vi "PSTR-Replot PSDs.vi"(0 "Data":T1, 2 "Graph Ref":refnum<vi>, 5 "ifreq":i32, 9 "ilevel":i32, 11 "error in (no error)":errorcluster) -> (15 "error out":errorcluster)   [LabVIEW 2020]
uses:
  Typedefs/PSTR-Data.ctl
  Typedefs/PSTR-Model Fit.ctl
  Typedefs/PSTR-Fit Parameters.ctl
  epl-vi-lib/Utility VIs/Conversion VIs/Create Waveform Cluster (1D).vi
panel:
  # "NF x NL x 2 x Npts"
  # "NF x NL x Npts"
  # "NF x NL"
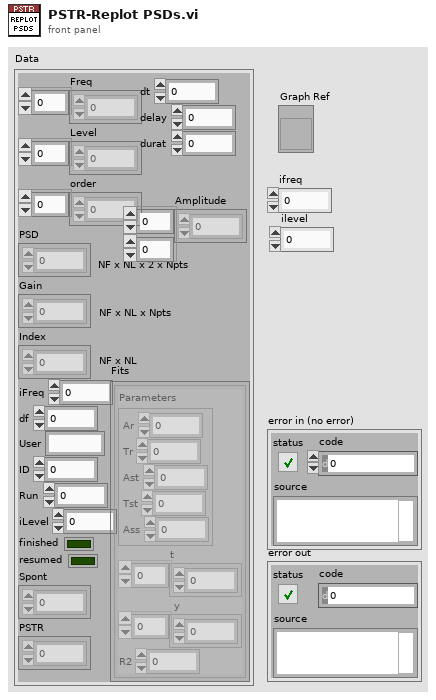
[diagram p1: front panel]
types:
  T1 = typedef "PSTR-Data.ctl" = cluster{"Freq":dbl[], "Level":dbl[], "order":i32[], "PSD":dbl[][][][], "Gain":dbl[][][], "Index":dbl[][], "iFreq":i32, "df":dbl, "User":string, "ID":i32, "Run":i32, "iLevel":i32, "finished":bool, "resumed":bool, "Spont":dbl[][], "PSTR":dbl[][][], "dt":dbl, "delay":dbl, "durat":dbl, "Fits":T2[][], "Amplitude":dbl[][]}
  T2 = typedef "PSTR-Model Fit.ctl" = cluster{"Parameters":T3, "t":dbl[], "y":dbl[], "R2":dbl}
  T3 = typedef "PSTR-Fit Parameters.ctl" = cluster{"Ar":dbl, "Tr":dbl, "Ast":dbl, "Tst":dbl, "Ass":dbl}
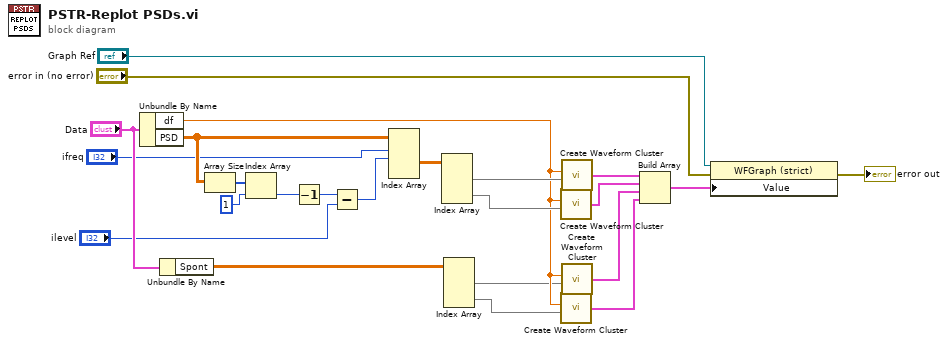
[diagram p0: block diagram]
diagram:
  n1 = Unbundle By Name("Data") -> ("df"=w15:dbl, "PSD"=w17:dbl[][][][])
  n2 = Unbundle By Name("Data") -> ("Spont"=w8:dbl[][])
  n3 = Array Size(array=w17) -> (size(s)=w23:i32[])
  n4 = Index Array(array=w23, index=1) -> (element=w3:i32)
  n5 = Decrement(x=w3) -> (x-1=w6:i32)
  n6 = Subtract(x=w6, y="ilevel") -> (x-y=w4:i32)
  n7 = Index Array(array=w17, index (dim 0)="ifreq", index (dim 1)=w4) -> (element=w22:dbl[][])  [unwired: 2 in]
  n8 = Index Array(array=w22) -> (element #1=w19:dbl[], element #2=w18:dbl[])  [unwired: 4 in]
  n9 = Index Array(array=w8) -> (element #1=w1:dbl[], element #2=w16:dbl[])  [unwired: 4 in]
  n10 = call-poly "Create Waveform Cluster.vi"("dx"=w15, "Y"=w18) -> ("waveform cluster"=w20:cluster{dbl, "dx":dbl, "Y":dbl[]})  [unwired: 3 in]
  n11 = call-poly "Create Waveform Cluster.vi"("dx"=w15, "Y"=w16) -> ("waveform cluster"=w13:cluster{dbl, "dx":dbl, "Y":dbl[]})  [unwired: 3 in]
  n12 = call-poly "Create Waveform Cluster.vi"("dx"=w15, "Y"=w19) -> ("waveform cluster"=w21:cluster{dbl, "dx":dbl, "Y":dbl[]})  [unwired: 3 in]
  n13 = call-poly "Create Waveform Cluster.vi"("dx"=w15, "Y"=w1) -> ("waveform cluster"=w14:cluster{dbl, "dx":dbl, "Y":dbl[]})  [unwired: 3 in]
  n14 = Build Array(w21, w20, w14, w13) -> (w12:cluster{dbl, "dx":dbl, "Y":dbl[]}[])
  n15 = property class="WFGraph (strict)"(reference="Graph Ref", error in="error in (no error)", "Value"=w12) -> (error out=→"error out":errorcluster)  [unwired: 1 out]
